vi "get data definition.vi"(10 "channel classification":T1, 11 "GPIC ScaleAndLimit runtime in":refnum<class "GPIC ScaleAndLimit runtime.lvclass">) -> (1 "valid?":bool, 2 "index cluster":variant, 3 "GPIC ScaleAndLimit runtime out":refnum<class "GPIC ScaleAndLimit runtime.lvclass">)   [LabVIEW 2015, in "GPIC ScaleAndLimit runtime.lvclass"]
uses:
  GPIC ScaleAndLimit runtime.lvclass
  <vilib>/NI/Tag Bus Module Framework/channel/channel classification.ctl
  input user data.ctl
  output user data.ctl
  parameter user data.ctl
  result user data.ctl
  <vilib>/NI/Tag Bus Module Framework/channel/TBM channel.lvclass
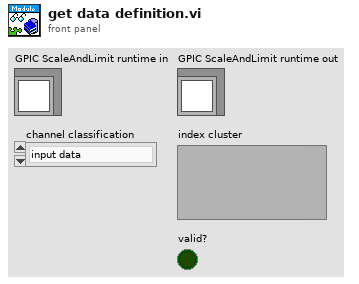
[diagram p1: front panel]
types:
  T1 = typedef "TBM channel.lvclass/channel classification.ctl" = enum16{"input data", "output data", "processing parameter", "processing result"}
  T2 = typedef "GPIC ScaleAndLimit runtime.lvclass/input user data.ctl" = cluster{"RMC/Simultaneous/AI0":sgl, "RMC/Simultaneous/AI1":sgl, "RMC/Simultaneous/AI2":sgl, "RMC/Simultaneous/AI3":sgl, "RMC/Simultaneous/AI4":sgl, "RMC/Simultaneous/AI5":sgl, "RMC/Simultaneous/AI6":sgl, "RMC/Simultaneous/AI7":sgl, "RMC/Simultaneous/AI8":sgl, "RMC/Simultaneous/AI9":sgl, "RMC/Simultaneous/AI10":sgl, "RMC/Simultaneous/AI11":sgl, "RMC/Simultaneous/AI12":sgl, "RMC/Simultaneous/AI13":sgl, "RMC/Simultaneous/AI14":sgl, "RMC/Simultaneous/AI15":sgl, "AILimits":bool, "AILimitHigh":u16, "AILimitLow":u16}
  T3 = typedef "GPIC ScaleAndLimit runtime.lvclass/output user data.ctl" = cluster{"ClearLimits":bool}
  T4 = typedef "GPIC ScaleAndLimit runtime.lvclass/parameter user data.ctl" = cluster{"fmwk_placeholder":i32}
  T5 = typedef "GPIC ScaleAndLimit runtime.lvclass/result user data.ctl" = cluster{"fmwk_placeholder":i32}
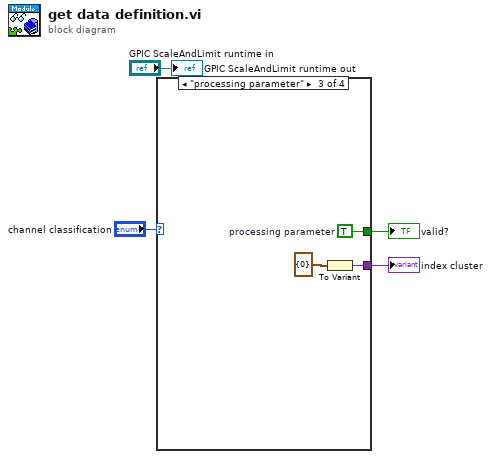
[diagram p0: block diagram]
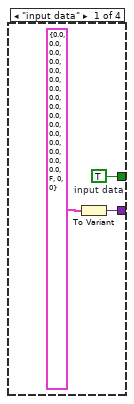
[diagram p2: hidden frame]
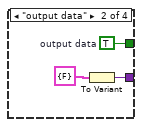
[diagram p3: hidden frame]
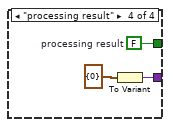
[diagram p4: hidden frame]
diagram:
  n1 = case shown="\"processing parameter\"" "channel classification" {
    tunnel: [w6 w10 w13 w16] -> w2
    tunnel: [w5 w9 w12 w15] -> w1
    frame "input data" {
      w5 = TRUE  # input data
      n2 = To Variant(anything=T2 {"RMC/Simultaneous/AI0"=0.0, "RMC/Simultaneous/AI1"=0.0, "RMC/Simultaneous/AI2"=0.0, "RMC/Simultaneous/AI3"=0.0, "RMC/Simultaneous/AI4"=0.0, "RMC/Simultaneous/AI5"=0.0, "RMC/Simultaneous/AI6"=0.0, "RMC/Simultaneous/AI7"=0.0, "RMC/Simultaneous/AI8"=0.0, "RMC/Simultaneous/AI9"=0.0, "RMC/Simultaneous/AI10"=0.0, "RMC/Simultaneous/AI11"=0.0, "RMC/Simultaneous/AI12"=0.0, "RMC/Simultaneous/AI13"=0.0, "RMC/Simultaneous/AI14"=0.0, "RMC/Simultaneous/AI15"=0.0, "AILimits"=FALSE, "AILimitHigh"=0, "AILimitLow"=0} ("Inputs from system")) -> (Variant=w6:variant)
    }
    frame "output data" {
      w9 = TRUE  # output data
      n3 = To Variant(anything=T3 {"ClearLimits"=FALSE} ("Outputs to system")) -> (Variant=w10:variant)
    }
    frame "processing parameter" {
      w12 = TRUE  # processing parameter
      n4 = To Variant(anything=T4 {"fmwk_placeholder"=0} ("Parameters to process")) -> (Variant=w13:variant)
    }
    frame "processing result" {
      w15 = FALSE  # processing result
      n5 = To Variant(anything=T5 {"fmwk_placeholder"=0} ("Results from processing")) -> (Variant=w16:variant)
    }
  }
  "index cluster" <- w2
  "valid?" <- w1
  "GPIC ScaleAndLimit runtime out" <- "GPIC ScaleAndLimit runtime in"
